vi "Run Test.vi"(8 "error in (no error)":errorcluster, 11 "Parallel Test In":refnum<class "Parallel Test.lvclass">) -> (0 "error out":errorcluster, 2 "Tests Passed":bool[](array[boolean]), 3 "Parallel Test Out":refnum<class "Parallel Test.lvclass">)   [LabVIEW 2015, in "Parallel Test.lvclass"]
uses:
  Parallel Test.lvclass
  typedefs/Parallel Return -- Cluster.ctl
  Test Class/Test Class.lvclass/Test Class.ctl
  <userlib>/_OpenG.lib/array/array.llb/Filter 1D Array with Scalar (Boolean)__ogtk.vi
  Test Class/Test Class.lvclass
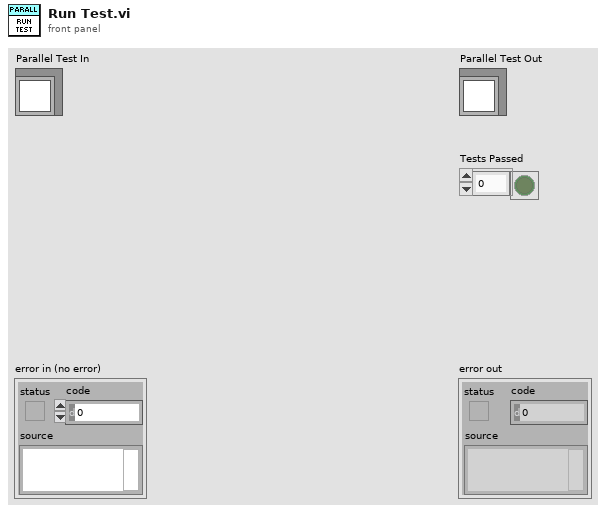
[diagram p1: front panel]
types:
  T1 = typedef "Parallel Test.lvclass/Parallel Return -- Cluster.ctl" = cluster{"Status":bool[], "Code":i32, "Source":string, "Position":u32[]}
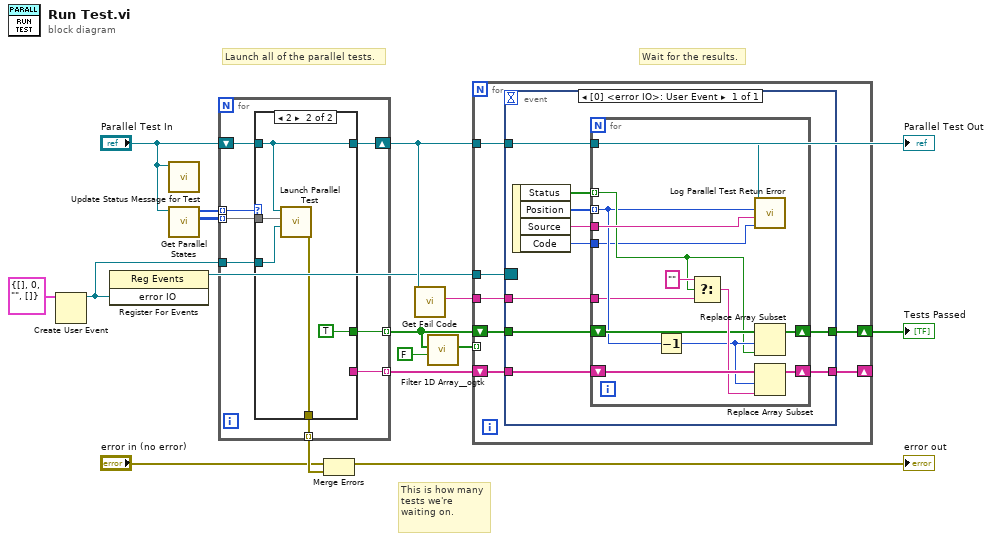
[diagram p0: block diagram]
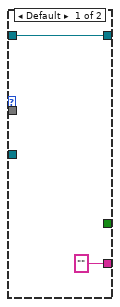
[diagram p2: hidden frame]
diagram:
  # "This is how many tests we're waiting on."
  # "Wait for the results."
  # "Launch all of the parallel tests."
  n1 = Create User Event(user event datatype=T1 {"Status"=[], "Code"=0, "Source"="", "Position"=[]} ("error IO")) -> (user event=w2:refnum<user-event>)  [unwired: 1 in, 1 out]
  n2 = register-events(w2) -> (reference out=w1:refnum<event-registration>)  [unwired: 2 in, 1 out]
  n3 = call-dynamic "Update Status Message for Test.vi"("Parallel Test in"="Parallel Test In") -> ()  [unwired: 11 in]
  n4 = call-dynamic "Get Parallel States.vi"("Parallel Test in"="Parallel Test In") -> ("Positions"=w6:u32[][], "States"=w7:u32[])  [unwired: 9 in]
  n5 = for {
    shift-right: [w20] -> w5
    shift-left: "Parallel Test In" -> [w24]
    tunnel: [w23] -> w12 mode=indexing
    tunnel: [w22] -> w14 mode=indexing
    tunnel: [w21] -> w13 mode=indexing
    tunnel: w7 -> [w19] mode=indexing
    tunnel: w6 -> [w18] mode=indexing
    tunnel: w2 -> [w17]
    n6 = case shown="2" w19 {
      tunnel: w24 -> [w26 w28]
      tunnel: [w26 w28] -> w20
      tunnel: w18 -> [_ w31]
      tunnel: w17 -> [_ w27]
      tunnel: [_ TRUE] -> w23
      tunnel: ["" _] -> w22
      tunnel: [_ w29] -> w21
      frame Default {
      }
      frame 2 {
        n7 = call "Launch Parallel Test.vi"("Test Complete Event"=w27, "Positions"=w31, "Parallel Test in"=w28) -> ("error out"=w29:errorcluster)  [unwired: 8 in]
      }
    }
  }
  "Parallel Test Out" <- w5
  n8 = Merge Errors("error in (no error)", w13) -> (→"error out":errorcluster)
  n9 = call "Get Fail Code.vi"("Test Class in"=w5) -> ("Fail Code"=w4:string)  [unwired: 9 in, 1 out]
  n10 = call-poly <userlib>:"Filter 1D Array__ogtk.vi"("items to filter"=FALSE, "array"=w12) -> ("filtered array"=w11:bool[])  [unwired: 4 in, 1 out]
  n11 = for {
    shift-right: [w36] -> w16
    shift-left: w12 -> [w38]
    shift-right: [w35] -> _
    shift-left: w14 -> [w37]
    tunnel: w11 -> [_] mode=indexing
    tunnel: w5 -> [w34]
    tunnel: w4 -> [w33]
    tunnel: w1 -> [w32]
    n12 = event shown="[0] <error IO>: User Event" {
      selector: w32 -> [_]
      dyn-events: _ -> [_]
      timeout: _ -> [_]
      tunnel: w34 -> [w40]
      tunnel: w38 -> [w46]
      tunnel: w37 -> [w47]
      tunnel: [w44] -> w36
      tunnel: [w43] -> w35
      tunnel: w33 -> [w39]
      event User Event {
        n13 = event-data() -> ("Status"=w45:bool[], "Position"=w42:u32[], "Source"=w48:string, "Code"=w41:i32)  [unwired: 1 in]
        n14 = for {
          tunnel: w48 -> [w60]
          tunnel: w45 -> [w55] mode=indexing
          tunnel: w42 -> [w52] mode=indexing
          tunnel: w41 -> [w51]
          tunnel: w40 -> [w50]
          tunnel: w39 -> [w49]
          shift-right: [w53] -> w43
          shift-left: w47 -> [w59]
          shift-right: [w54] -> w44
          shift-left: w46 -> [w57]
          n15 = Decrement(x=w52) -> (x-1=w56:u32)
          n16 = Select(t="", s=w55, f=w49) -> (s? t:f=w58:string)
          n17 = call "Log Parallel Test Retun Error.vi"("code"=w51, "source"=w60, "Position"=w52, "Parallel Test"=w50) -> ()  [unwired: 8 in]
          n18 = Replace Array Subset(array=w57, new element=w55, index=w56) -> (w54:bool[])
          n19 = Replace Array Subset(array=w59, new element=w58, index=w56) -> (w53:string[])
        }
      }
    }
  }
  "Tests Passed" <- w16
